vi "slow_control_alpha.vi"() -> ()   [LabVIEW 2018]
uses:
  <instrlib>/Lake Shore 335/Lake Shore 335.lvlib
  <instrlib>/CAEN PSM/CAEN PSM.lvlib
panel:
  in  "stop":bool
  out "Anode resets in":string
  out "CAEN 1 \nVoltages":dbl[](array[numeric])
  out "Started up?":bool
  out "Try 2 Inside loop":dbl[][](array[numeric])
  in  "Read T every N cycles":i32=2
  out "Time until next cycle":dbl
  in  "Time per cycle (s)":i32=2 caption="Time Target (s)"
  in  "input cluster":errorcluster
  in  "Allows tabs on \nfront panel":T1(tab)
  in  "COM-port NI-box":refnum<visa-resource-name>
  in  "COM-port LakeShore":refnum<visa-resource-name>
  in  "ID Query":bool=TRUE
  in  "COM-port CAEN 1":refnum<visa-resource-name>
  in  "COM-port CAEN 2":refnum<visa-resource-name>
  in  "Ignore Initialization Errors":bool caption="Ignore init. errors?"
  out "LakeShore status":bool
  out "NI-box status":bool
  out "CAEN 1 status":bool
  out "CAEN 2 status":bool
  out "Initialization status":bool
  in  "VSet":dbl[](array[numeric])
  in  "IMax (uA)":dbl[](array[numeric])
  in  "VMax (V)":dbl[](array[numeric])
  out "Cathode":dbl(knob) scale=0.0..5000.0
  out "Anode":dbl(knob) scale=0.0..4000.0
  out "PMT 2":dbl(knob) scale=0.0..1000.0
  out "PMT 1":dbl(knob) scale=1.0..1000.0
  in  "Read V every N cycles":i16=120
  out "CAEN 1\nVmon (V)":dbl[](array[numeric])
  out "CAEN 1\nIMon (uA)":dbl[](array[numeric])
  in  "Reset anode":bool=TRUE
  in  "Kill every Y minutes":i32
  in  "Keep off for X seconds":i32
  out "Total cycles in Anode Reset Routine":i32
  out "Current modulated cycle number":i32
  out "VSet killed":bool
  out "VSet applied":bool
  # "<- Proof of concept for New/Old T + New P"
  # "PMT 1"
  # "PMT 2"
  # "Anode"
  # "Cathode"
  # "seconds"
  # "Connection settings"
  # "Lakeshore settings"
  # "Pressure correction settings"
  # "Pressure correction factors go here.\nPrecisely, offsets and multiplication factors\nin the voltages passed from the pressure-\nsensors to the NI-box."
  # "Might need to split up NI-box com port.\nPreferable to task it with measuring T\nand P seperately.\nPerhaps need to set task per single channel."
  # "Alarm indicators"
  # "CAEN 1"
  # "Data"
  # "PMT 1"
  # "PMT 1"
  # "PMT 2"
  # "PMT 2"
  # "Arrays from CAEN 2 go here"
  # "Anode"
  # "Anode"
  # "Cathode"
  # "Cathode"
  # "Settings"
  # "CAEN 1"
  # "CAEN 2"
  # "PMT 1"
  # "PMT 2"
  # "Anode"
  # "CAEN 2"
  # "Cathode"
  # "PMT 1"
  # "PMT 2"
  # "Anode"
  # "Cathode"
  # "Needle gauges or other displays go here"
  # "PMT 1"
  # "PMT 2"
  # "Anode"
  # "Cathode"
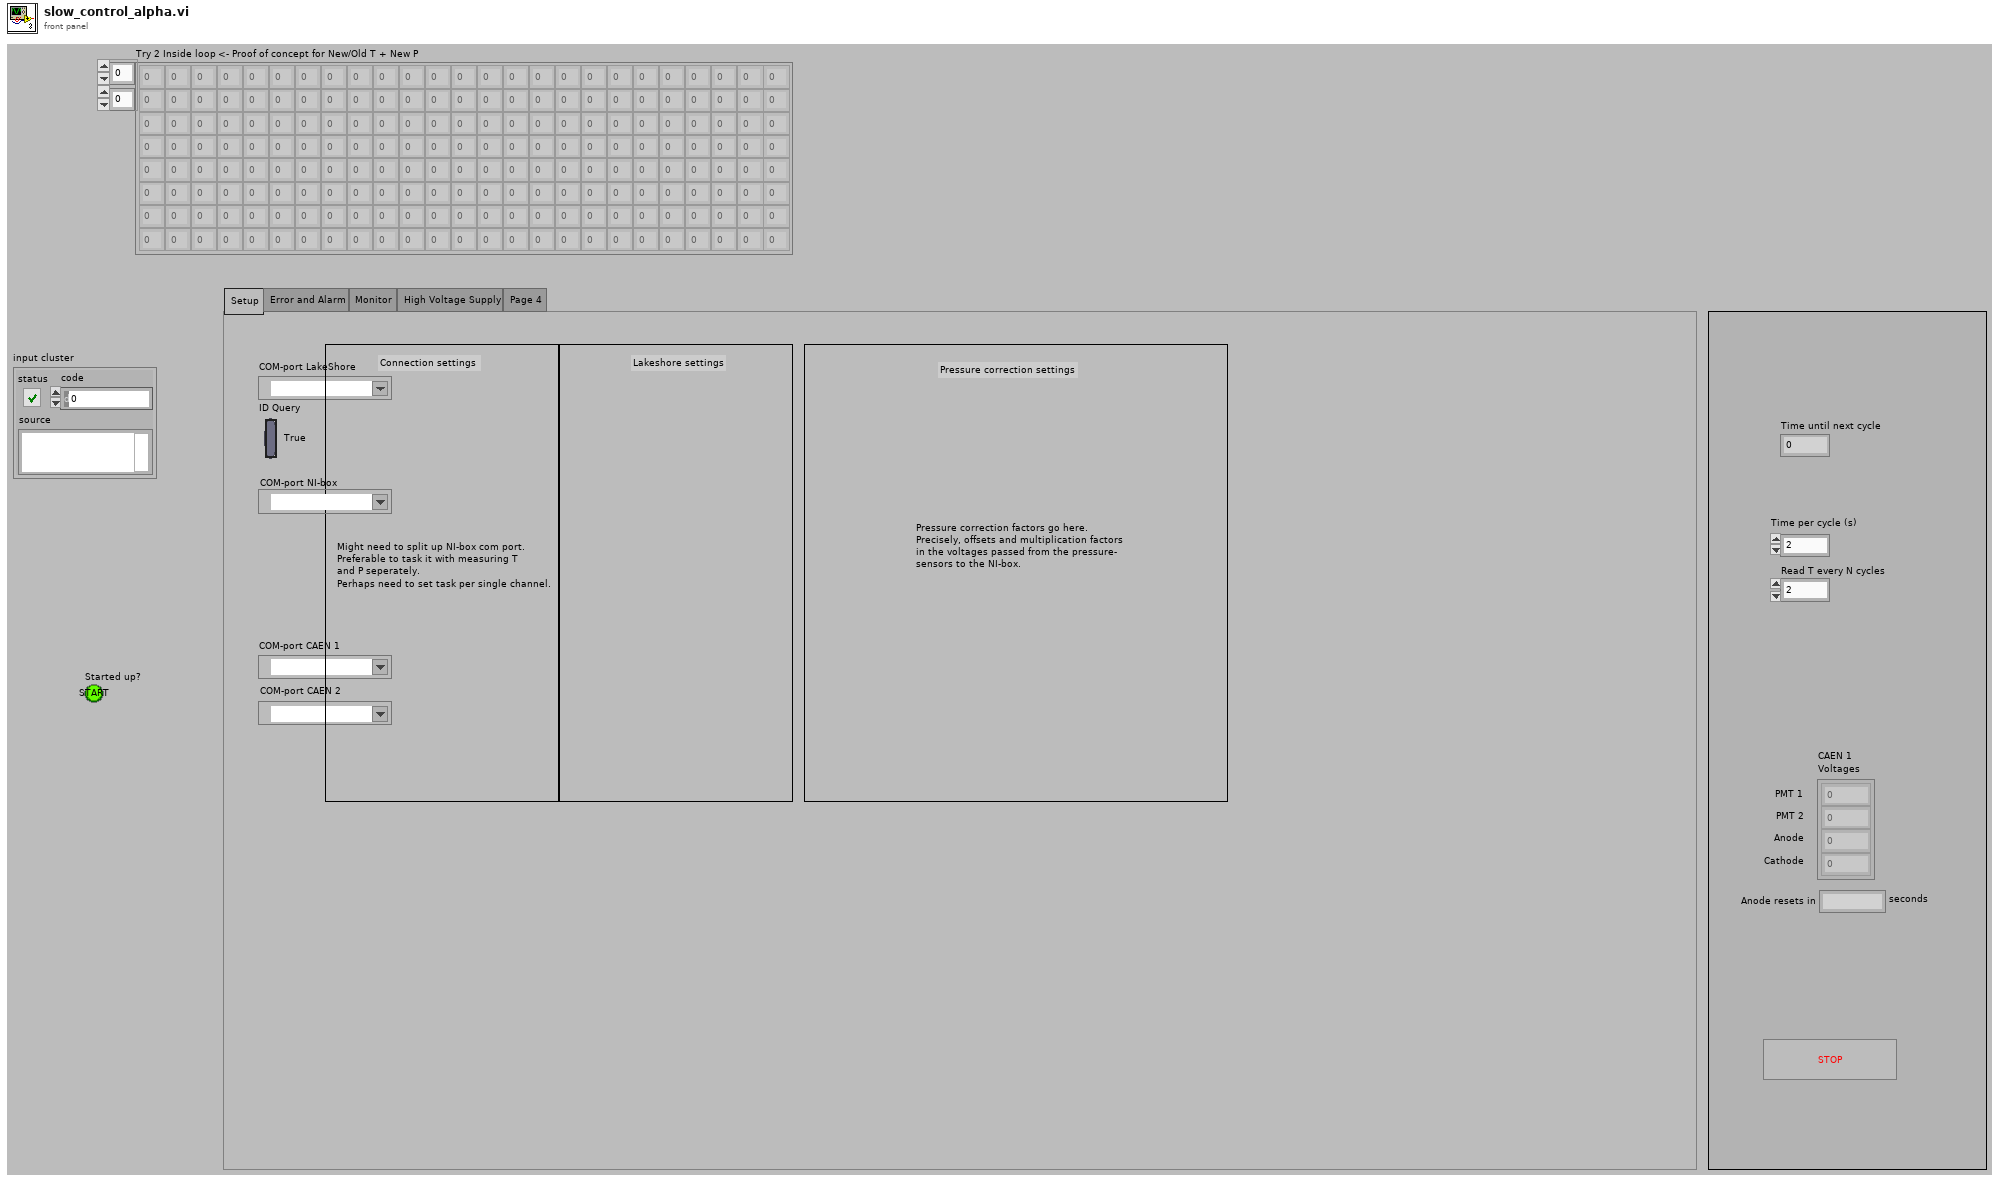
[diagram p1: front panel]
types:
  T1 = enum32{"Setup", "Error and Alarm", "Monitor", "High Voltage Supply", "Page 4"}
  T2 = cluster{"Flow Control":u16, "Stop Bits":u16, "Data Bits":u16, "Parity":u16, "Baud Rate":u32}
  T3 = cluster{"VISA resource name out":refnum<visa-resource-name>, "error out":errorcluster}
  T4 = cluster{"VMax (V)":dbl[], "IMax (uA)":dbl[], "VSet":dbl[]}
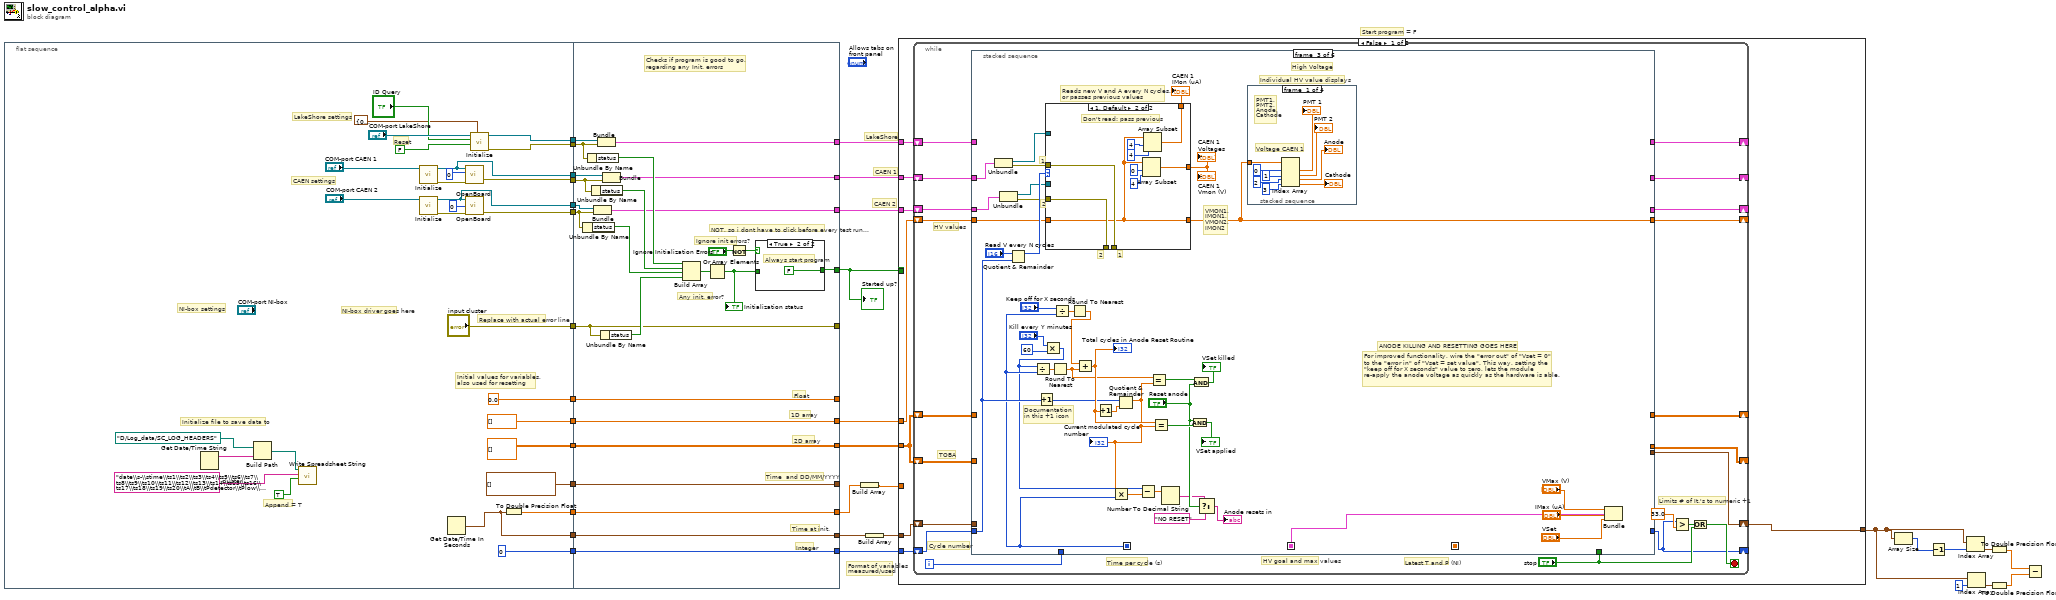
[diagram p0: block diagram]
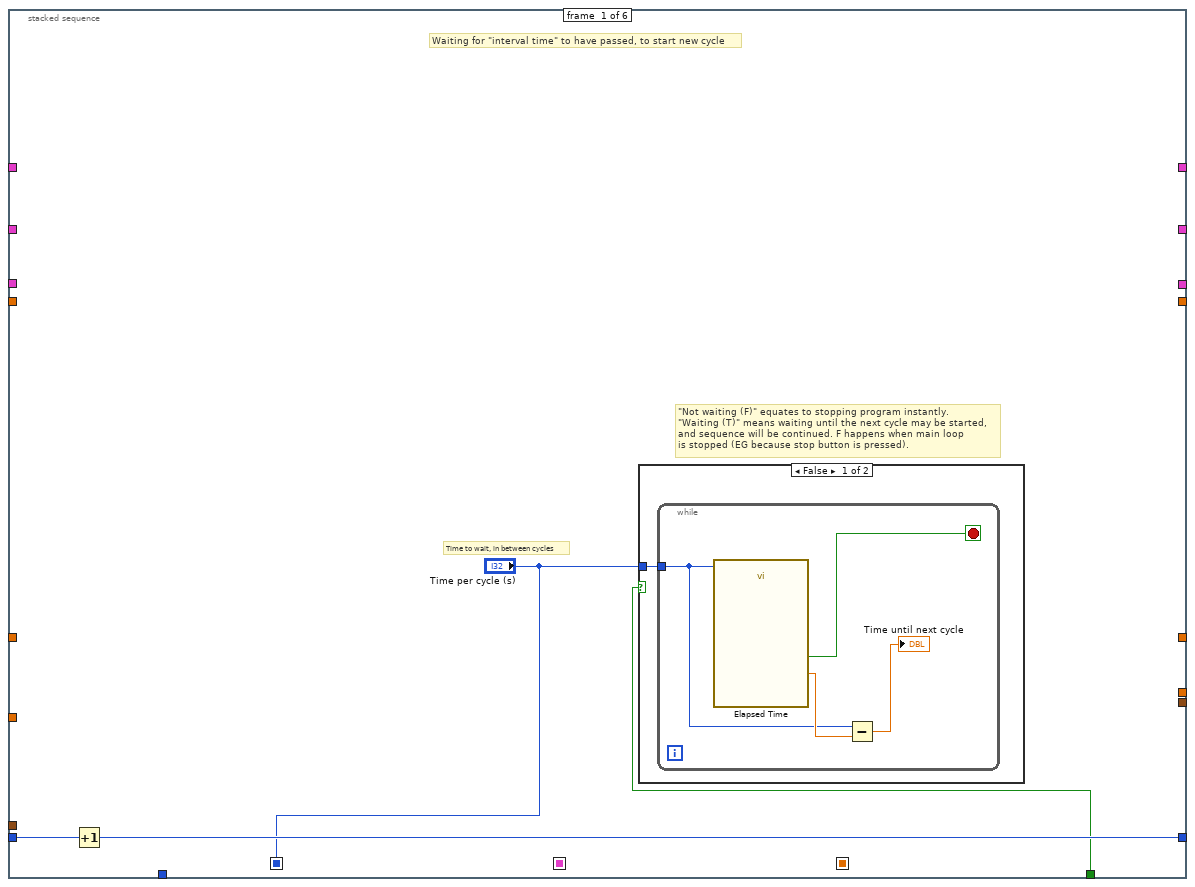
[diagram p2: hidden frame]
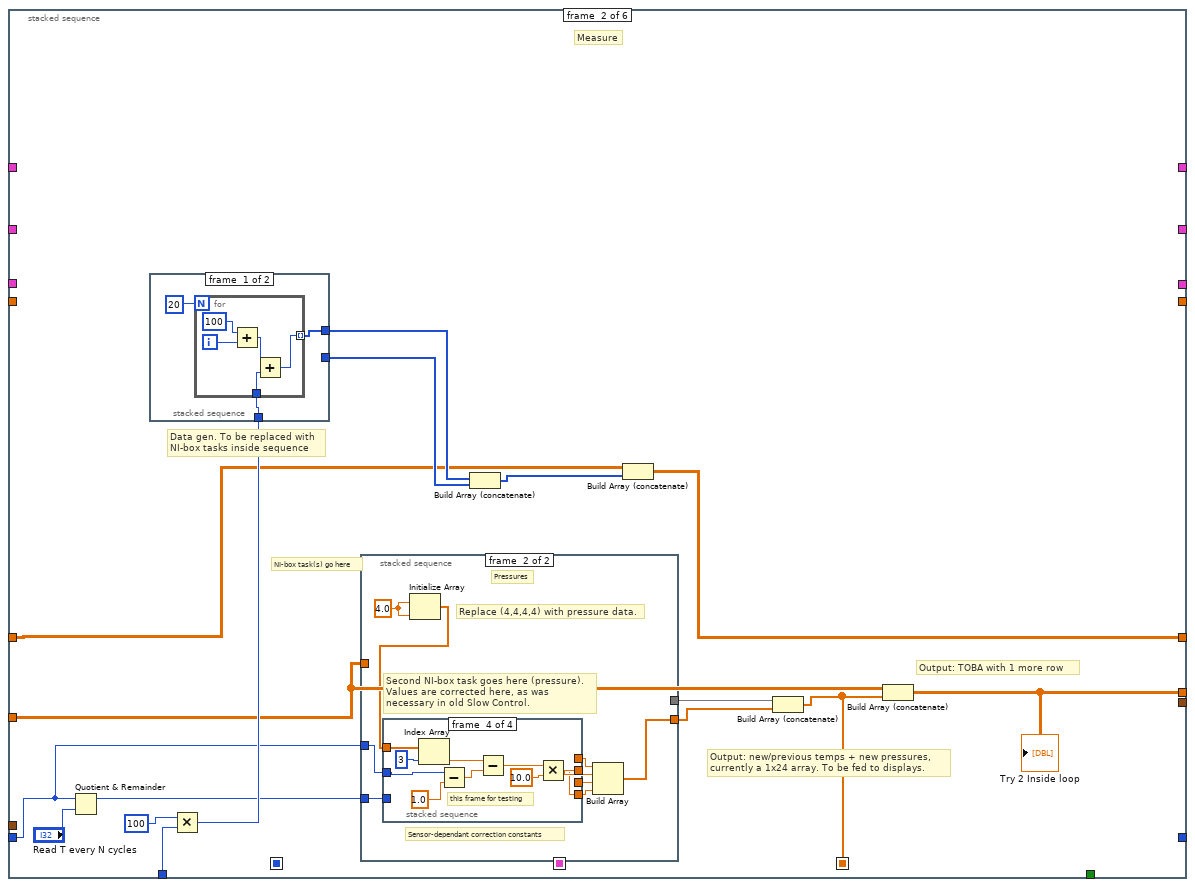
[diagram p4: hidden frame]
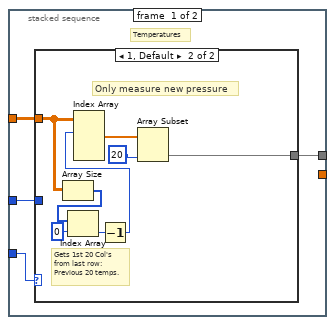
[diagram p5: hidden frame]
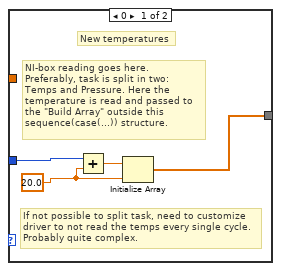
[diagram p6: hidden frame]
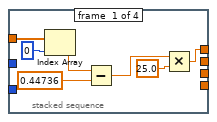
[diagram p7: hidden frame]
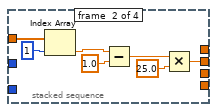
[diagram p8: hidden frame]
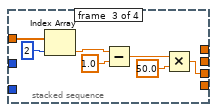
[diagram p9: hidden frame]
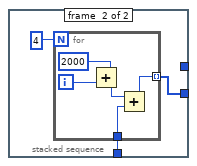
[diagram p10: hidden frame]
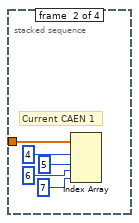
[diagram p11: hidden frame]
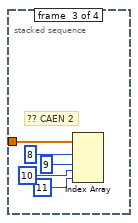
[diagram p12: hidden frame]
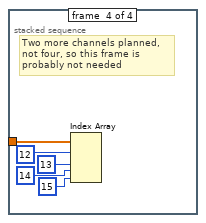
[diagram p13: hidden frame]
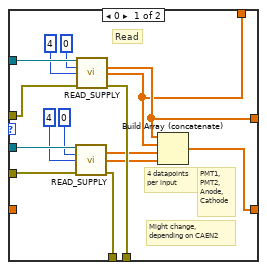
[diagram p14: hidden frame]
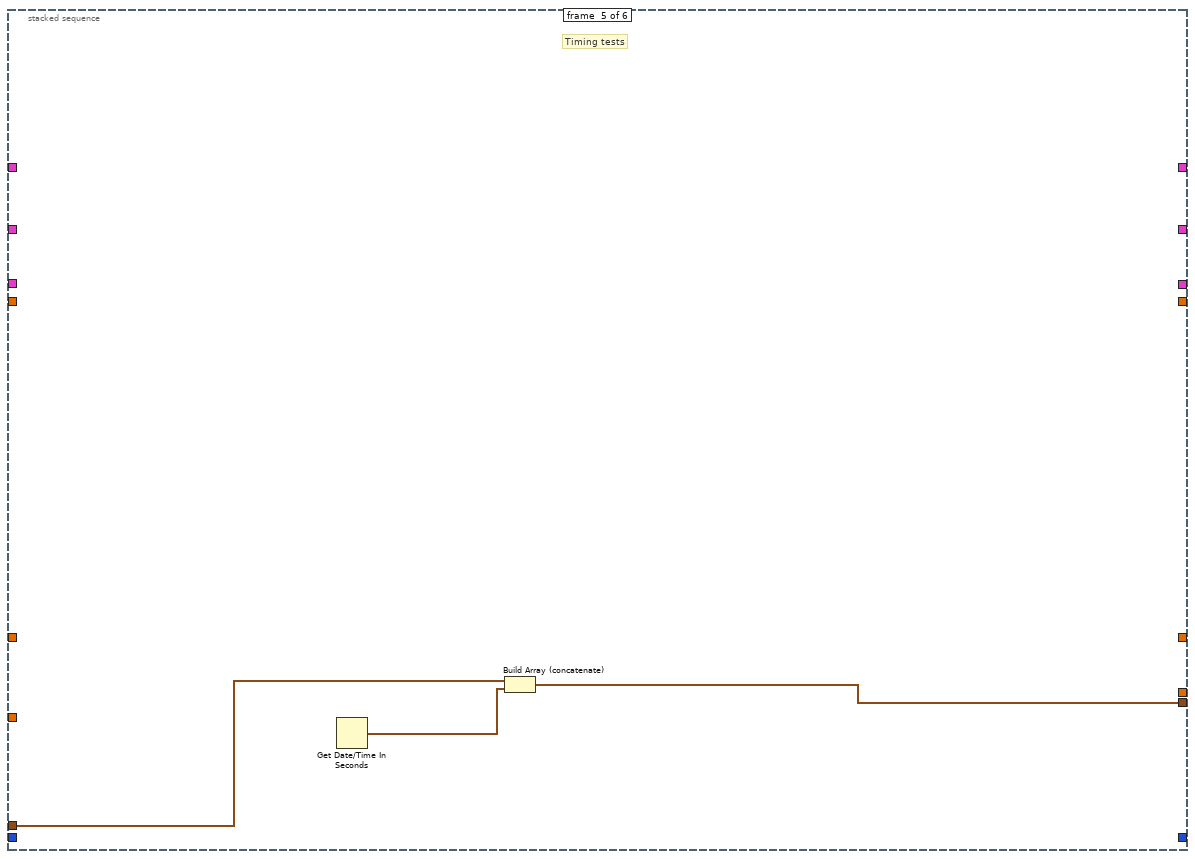
[diagram p16: hidden frame]
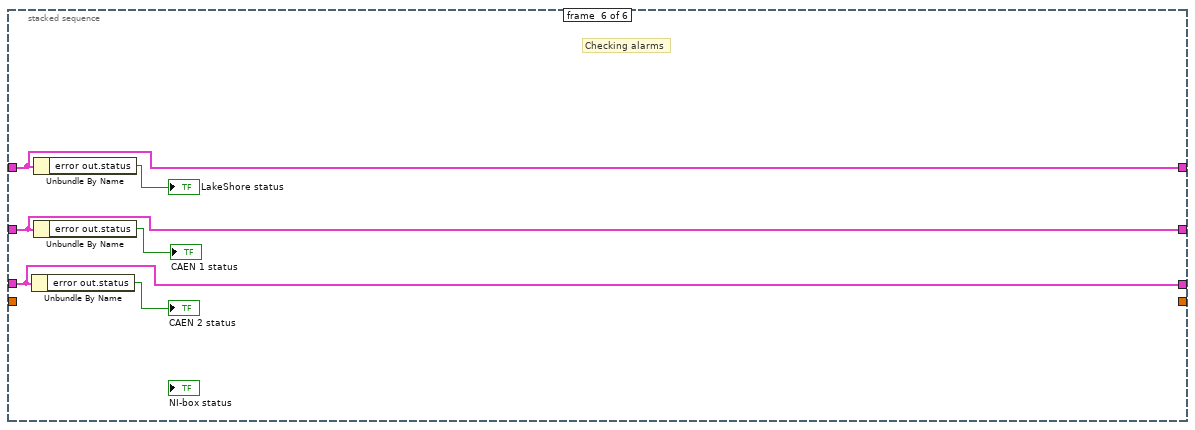
[diagram p17: hidden frame]
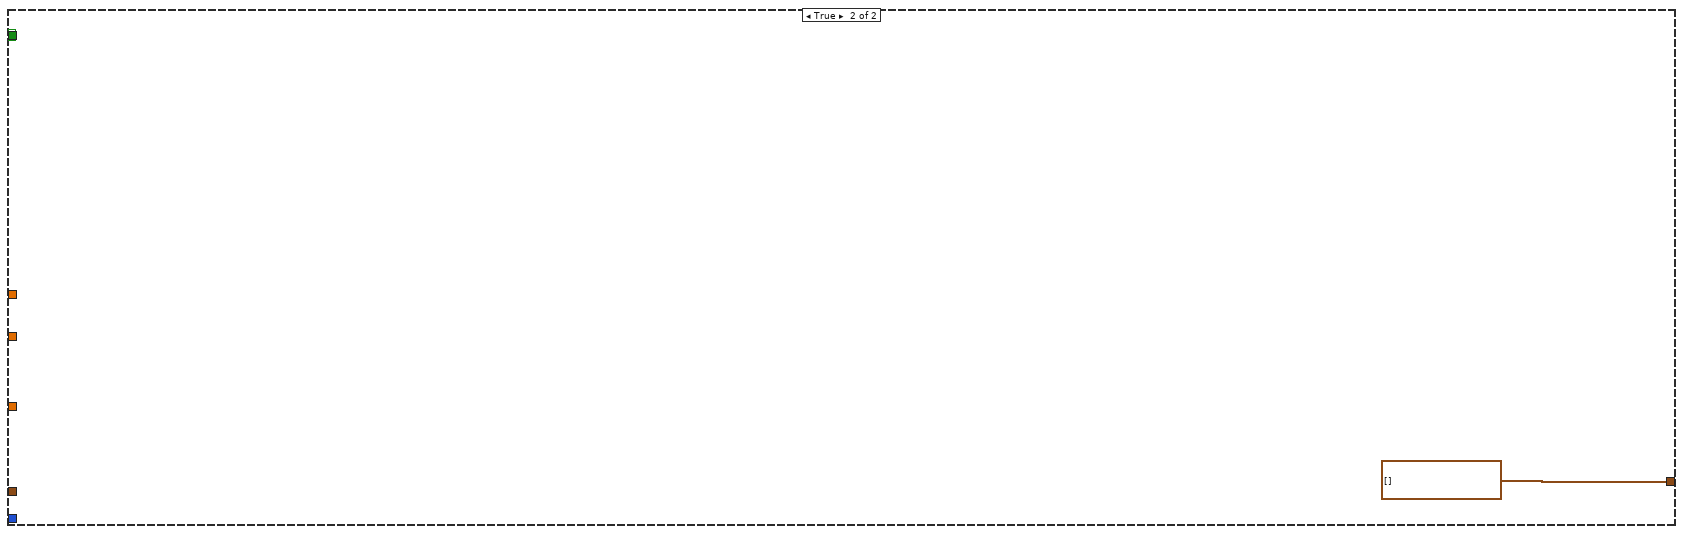
[diagram p18: hidden frame]
diagram:
  # "Start program = F"
  # "CAEN 2"
  # "CAEN 1"
  # "LakeShore"
  # "Format of variables\nmeasured/used"
  n1 = flat-sequence {
    tunnel: [w59] -> w33
    tunnel: [w58] -> w32
    tunnel: [w54] -> w31
    tunnel: [w53] -> w30
    tunnel: ["input cluster"] -> w29
    tunnel: [0.0] -> w28
    tunnel: [dbl[] []] -> w27
    tunnel: [dbl[][] []] -> w26
    tunnel: [timestamp[] []] -> w25
    tunnel: [0] -> w24
    tunnel: [w46] -> w23
    tunnel: [w39] -> w15
    tunnel: [w35] -> w4
    tunnel: [w34] -> w3
    tunnel: w33 -> [w75]
    tunnel: w32 -> [w74]
    tunnel: w31 -> [w72]
    tunnel: w30 -> [w71]
    tunnel: w29 -> [w77]
    tunnel: [w84] -> w1
    tunnel: [w82] -> _
    tunnel: w28 -> [w82]
    tunnel: [w81] -> w22
    tunnel: w27 -> [w81]
    tunnel: [w80] -> w20
    tunnel: w26 -> [w80]
    tunnel: [w79] -> _
    tunnel: w25 -> [w79]
    tunnel: [w78] -> w21
    tunnel: w24 -> [w78]
    tunnel: [w77] -> _
    tunnel: [w76] -> w17
    tunnel: w23 -> [w76]
    tunnel: [w73] -> w19
    tunnel: [w70] -> w18
    tunnel: [w67] -> w14
    tunnel: w15 -> [w67]
    tunnel: w4 -> [w65]
    tunnel: w3 -> [w64]
    tunnel: [w63] -> w2
    frame #0 {
      # "Append = T"
      # "Change to fit order of data in cluster"
      # "Initialize file to save data to"
      # "Initial values for variables,\nalso used for resetting"
      # "Replace with actual error line"
      # "NI-box driver goes here"
      # "NI-box settings"
      # "CAEN settings"
      # "Reset"
      # "LakeShore settings"
      n2 = Get Date/Time String() -> (date string=w42:string)  [unwired: 3 in, 1 out]
      n3 = Build Path(base path=path "D:/Log_data/SC_LOG_HEADERS", name or relative path=w42) -> (appended path=w45:path)
      n4 = call <vilib>:"Write Spreadsheet String.vi"("append to file? (new file:F)"=TRUE, "spreadsheet string"="date\\s-\\stime\\ts1\\ts2\\ts3\\ts4\\ts5\\ts6\\ts7\\ts8\\ts9\\ts10\\ts11\\ts12\\ts13\\ts14\\ts15\\ts16\\ts17\\ts18\\ts19\\ts20\\tA\\tB\\tPdetector\\tPlow\\tPhigh\\tFlow\\tHeater\\tSetpoint\\tCapacitance\\tTimestamp\\tInterval\\tLevel\\tV_PMT1\\tV_PMT2\\tV_Anode\\tV_cathode\\tI_PMT1\\tI_PMT2\\tI_Anode\\tI_cathode\\t\\r\\n", "file path (dialog if empty)"=w45) -> ()  [unwired: 7 in, 2 out]
      n5 = call <instrlib>:"Initialize.vi"("VISA resource name"="COM-port CAEN 1") -> ("error out"=w55:errorcluster, "VISA resource name out"=w54:refnum<visa-resource-name>)  [unwired: 9 in]
      n6 = call <instrlib>:"Initialize.vi"("VISA resource name"="COM-port CAEN 2") -> ("error out"=w36:errorcluster, "VISA resource name out"=w35:refnum<visa-resource-name>)  [unwired: 9 in]
      n7 = Get Date/Time In Seconds() -> (seconds since 1Jan1904=w39:timestamp)
      n8 = call <instrlib>:"OpenBoard.vi"("error in (no error)"=w55, "Board Address"=0, "VISA resource name"=w54) -> ("error out"=w53:errorcluster)  [unwired: 7 in, 1 out]
      n9 = call <instrlib>:"OpenBoard.vi"("error in (no error)"=w36, "Board Address"=u8 0, "VISA resource name"=w35) -> ("error out"=w34:errorcluster)  [unwired: 7 in, 1 out]
      n10 = call <instrlib>:"Initialize.vi"("Serial Configuration"=T2 {"Flow Control"=0, "Stop Bits"=10, "Data Bits"=7, "Parity"=1, "Baud Rate"=57600}, "Reset (True)"=FALSE ("Reset (LakeShore)"), "ID Query (True)"="ID Query", "VISA resource name"="COM-port LakeShore") -> ("error out"=w58:errorcluster, "VISA resource name out"=w59:refnum<visa-resource-name>)  [unwired: 6 in]
      n11 = To Double Precision Float(number=w39) -> (double precision float=w46:dbl)
    }
    frame #1 {
      # "NOT, so i dont have to click before every test run..."
      # "Time at init."
      # "Integer"
      # "Time  and DD/MM/YYYY"
      # "2D array"
      # "1D array"
      # "Float"
      # "Checks if program is good to go,\nregarding any Init. errors"
      # "Ignore init errors?"
      # "Any init. error?"
      n12 = Unbundle By Name(w64) -> ("status"=w66:bool)
      n13 = Unbundle By Name(w74) -> ("status"=w85:bool)
      n14 = Unbundle By Name(w71) -> ("status"=w87:bool)
      n15 = Bundle("VISA resource name out"=w65, "error out"=w64) -> (w63:T3)  [unwired: 1 in]
      n16 = Bundle("VISA resource name out"=w75, "error out"=w74) -> (w73:T3)  [unwired: 1 in]
      n17 = Unbundle By Name(w77) -> ("status"=w86:bool)
      n18 = Bundle("VISA resource name out"=w72, "error out"=w71) -> (w70:T3)  [unwired: 1 in]
      n19 = Build Array(w85, w87, w86, w66) -> (w88:bool[])
      n20 = Or Array Elements(Boolean array=w88) -> (logical OR=w83:bool)
      "Initialization status" <- w83
      n21 = Not(x="Ignore Initialization Errors") -> (.not. x?=w68:bool)
      n22 = case shown="True" w68 {
        tunnel: [w89 FALSE] -> w84
        tunnel: w83 -> [w89 _]
        frame False {
          # "Only start if no errors"
        }
        frame True {
          # "Always start program"
        }
      }
    }
  }
  n23 = Build Array(w17) -> (w16:dbl[])
  n24 = Build Array(w14) -> (w13:timestamp[])
  n25 = case shown="False" w1 {
    selector: w1 -> [_ w314]
    tunnel: [_ w314] -> _
    tunnel: w22 -> [w93 _]
    tunnel: w21 -> [w98 _]
    tunnel: w20 -> [w97 _]
    tunnel: w19 -> [w91 _]
    tunnel: w18 -> [w94 _]
    tunnel: w16 -> [_ _]
    tunnel: w13 -> [w96 _]
    tunnel: [w95 timestamp[] []] -> w9
    tunnel: w2 -> [w92 _]
    frame False {
      n26 = while {
        shift-right: [w107] -> _
        shift-left: w98 -> [w119]
        shift-right: [w113] -> _
        shift-left: w97 -> [w112]
        shift-right: [w110] -> _
        shift-left: w97 -> [w111]
        shift-right: [w108] -> w95
        shift-left: w96 -> [w109]
        shift-right: [w101] -> _
        shift-left: w94 -> [w106]
        shift-right: [w99] -> _
        shift-left: w93 -> [w105]
        shift-right: [w100] -> _
        shift-left: w92 -> [w104]
        shift-right: [w102] -> _
        shift-left: w91 -> [w103]
        i -> [w114]
        stop <- w115 stop-if-true
        # "Time per cycle (s)"
        # "Cycle number"
        # "HV goal and max values"
        # "HV values"
        # "TOBA"
        # "Latest T and P (NI)"
        # "Limits # of It.'s to numeric +1"
        n27 = stacked-sequence {
          seq-local: [_ w131 _ _ _ _] -> [_ _ _ _ _ _]
          seq-local: [_ _ w240 _ _ _] -> [_ _ _ _ _ _]
          seq-local: ["Time per cycle (s)" _ _ _ _ _] -> [_ _ w218 _ _ _]
          tunnel: [w122 _ _ _ _ _] -> w107
          tunnel: "stop" -> [w121 _ _ _ _ _]
          tunnel: w119 -> [w123 w129 w235 _ _ _]
          tunnel: w114 -> [_ w130 _ _ _ _]
          tunnel: w112 -> [_ w136 _ _ _ _]
          tunnel: [_ w140 _ _ _ _] -> w113
          tunnel: w111 -> [_ w132 _ _ _ _]
          tunnel: [_ w133 _ _ _ _] -> w110
          tunnel: w109 -> [_ _ _ _ w305 _]
          tunnel: [_ _ _ _ w304 _] -> w108
          tunnel: w106 -> [_ _ w253 _ _ w309]
          tunnel: w105 -> [_ _ w250 _ _ _]
          tunnel: w104 -> [_ _ w249 _ _ w308]
          tunnel: w103 -> [_ _ _ _ _ w307]
          tunnel: [_ _ _ _ _ w307] -> w102
          tunnel: [_ _ _ _ _ w309] -> w101
          tunnel: [_ _ _ _ _ w308] -> w100
          tunnel: [_ _ w246 _ _ _] -> w99
          frame #0 {
            # "Time to wait, in between cycles"
            # "\"Not waiting (F)\" equates to stopping program instantly.\n\"Waiting (T)\" means waiting until the next cycle may be started,\nand sequence will be continued. F happens when main loop \nis stopped (EG because stop button is pressed)."
            # "Waiting for \"interval time\" to have passed, to start new cycle"
            n28 = Increment(x=w123) -> (x+1=w122:i32)
            n29 = case shown="False" w121 {
              tunnel: "Time per cycle (s)" -> [w124 _]
              frame False {
                n30 = while {
                  tunnel: w124 -> [w126]
                  stop <- w128 stop-if-true
                  n31 = call "Elapsed Time"("Time Target (s)"=w126) -> ("Elapsed Time (s)"=w127:dbl, "Time has Elapsed"=w128:bool)  [unwired: 11 in, 6 out]
                  n32 = Subtract(x=w126, y=w127) -> (x-y=→"Time until next cycle":dbl)
                }
              }
              frame True {
              }
            }
          }
          frame #1 {
            # "Output: TOBA with 1 more row"
            # "Output: new/previous temps + new pressures,\ncurrently a 1x24 array. To be fed to displays."
            # "NI-box task(s) go here"
            # "Data gen. To be replaced with\nNI-box tasks inside sequence"
            # "Measure"
            n33 = Quotient & Remainder(x=w129, y="Read T every N cycles") -> (x-y*floor(x/y)=w137:i32)  [unwired: 1 out]
            n34 = Multiply(x=100, y=w130) -> (x*y=w143:i32)
            n35 = stacked-sequence {
              tunnel: [w201 _] -> w142
              tunnel: [_ w209] -> w141
              tunnel: w143 -> [w200 w208]
              frame #0 {
                n36 = for {
                  N: 20 -> [_]
                  tunnel: [w203] -> w201 mode=indexing
                  tunnel: w200 -> [w205]
                  i -> [w206]
                  n37 = Add(x=100, y=w206) -> (x+y=w204:i32)
                  n38 = Add(x=w204, y=w205) -> (x+y=w203:i32)
                }
              }
              frame #1 {
                n39 = for {
                  N: 4 -> [_]
                  tunnel: [w212] -> w209 mode=indexing
                  tunnel: w208 -> [w211]
                  i -> [w214]
                  n40 = Add(x=2000, y=w214) -> (x+y=w213:i32)
                  n41 = Add(x=w213, y=w211) -> (x+y=w212:i32)
                }
              }
            }
            n42 = stacked-sequence {
              tunnel: w137 -> [w148 w162]
              tunnel: [w147 _] -> w135
              tunnel: [_ w165] -> w134
              tunnel: w132 -> [w146 _]
              tunnel: w129 -> [w145 w161]
              frame #0 {
                # "Temperatures"
                n43 = case shown="1, Default" w148 {
                  tunnel: w146 -> [_ w157]
                  tunnel: [w150 w153] -> w147
                  tunnel: w145 -> [w149 _]
                  frame 0 {
                    w151 = 20.0 ("element")
                    # "If not possible to split task, need to customize\ndriver to not read the temps every single cycle.\nProbably quite complex."
                    # "NI-box reading goes here.\nPreferably, task is split in two: \nTemps and Pressure. Here the \ntemperature is read and passed to \nthe \"Build Array\" outside this \nsequence(case(...)) structure."
                    # "New temperatures"
                    n44 = Add(x=w149, y=w151) -> (x+y=w152:dbl)
                    n45 = Initialize Array(w152, w151) -> (w150:dbl[])
                  }
                  frame 1, Default {
                    # "Gets 1st 20 Col's\nfrom last row:\nPrevious 20 temps."
                    # "Only measure new pressure"
                    n46 = Array Size(array=w157) -> (size(s)=w159:i32[])
                    n47 = Index Array(array=w159, index=0) -> (element=w160:i32)
                    n48 = Decrement(x=w160) -> (x-1=w156:i32)
                    n49 = Index Array(array=w157, index (row) #1=w156) -> (element #1=w155:dbl[])  [unwired: 3 in, 1 out]
                    n50 = Array Subset(array=w155, length=20) -> (w153:dbl[])  [unwired: 1 in]
                  }
                }
              }
              frame #1 {
                w164 = 4.0 ("element")
                # "Replace (4,4,4,4) with pressure data."
                # "Second NI-box task goes here (pressure).\nValues are corrected here, as was \nnecessary in old Slow Control."
                # "Sensor-dependant correction constants"
                # "Pressures"
                n51 = Initialize Array(w164, w164) -> (w163:dbl[])
                n52 = stacked-sequence {
                  tunnel: w163 -> [w171 w183 w190 w199]
                  tunnel: [w172 _ _ _] -> w169
                  tunnel: [_ w178 _ _] -> w168
                  tunnel: [_ _ w185 _] -> w167
                  tunnel: [_ _ _ w195] -> w166
                  tunnel: w162 -> [_ _ _ _]
                  tunnel: w161 -> [_ _ _ w191]
                  frame #0 {
                    n53 = Index Array(array=w171, index=0) -> (element=w170:dbl)
                    n54 = Subtract(x=w170, y=0.44736) -> (x-y=w174:dbl)
                    n55 = Multiply(x=w174, y=25.0) -> (x*y=w172:dbl)
                  }
                  frame #1 {
                    n56 = Index Array(array=w183, index=1) -> (element=w177:dbl)
                    n57 = Subtract(x=w177, y=1.0) -> (x-y=w180:dbl)
                    n58 = Multiply(x=w180, y=25.0) -> (x*y=w178:dbl)
                  }
                  frame #2 {
                    n59 = Index Array(array=w190, index=2) -> (element=w184:dbl)
                    n60 = Subtract(x=w184, y=1.0) -> (x-y=w187:dbl)
                    n61 = Multiply(x=w187, y=50.0) -> (x*y=w185:dbl)
                  }
                  frame #3 {
                    # "this frame for testing"
                    n62 = Index Array(array=w199, index=3) -> (element=w194:dbl)
                    n63 = Subtract(x=w191, y=1.0) -> (x-y=w192:dbl)
                    n64 = Subtract(x=w194, y=w192) -> (x-y=w197:dbl)
                    n65 = Multiply(x=w197, y=10.0) -> (x*y=w195:dbl)
                  }
                }
                n66 = Build Array(w169, w168, w167, w166) -> (w165:dbl[])
              }
            }
            n67 = Build Array (concatenate)(w142, w141) -> (w139:i32[])
            n68 = Build Array (concatenate)(w136, w139) -> (w140:dbl[][])
            n69 = Build Array (concatenate)(w135, w134) -> (w131:dbl[])
            n70 = Build Array (concatenate)(w132, w131) -> (w133:dbl[][])
            "Try 2 Inside loop" <- w133
          }
          frame #2 {
            # "VMON1, \nIMON1,\nVMON2,\nIMON2"
            # "For improved functionality, wire the \"error out\" of \"Vset = 0\"\nto the \"error in\" of \"Vset = set value\". This way, setting the\n\"keep off for X seconds\" value to zero, lets the module \nre-apply the anode voltage as quickly as the hardware is able."
            # "ANODE KILLING AND RESETTING GOES HERE"
            # "Documentation\nin this +1 icon"
            # "Individual HV value displays"
            # "1"
            # "2"
            # "1"
            # "2"
            # "Reads new V and A every N cycles,\nor passes previous values"
            # "High Voltage"
            n71 = Unbundle(w253) -> ("VISA resource name out"=w252:refnum<visa-resource-name>, "error out"=w251:errorcluster)
            n72 = Unbundle(w249) -> ("VISA resource name out"=w248:refnum<visa-resource-name>, "error out"=w247:errorcluster)
            n73 = Quotient & Remainder(x="Read V every N cycles", y=w235) -> (x-y*floor(x/y)=w254:i32)  [unwired: 1 out]
            n74 = Increment(x=w235) -> (x+1=w225:i32)
            n75 = Multiply(x="Kill every Y minutes", y=60) -> (x*y=w216:i32)
            n76 = Divide(x=w216, y=w218) -> (x/y=w228:dbl)
            n77 = case shown="1, Default" w254 {
              tunnel: w252 -> [w294 _]
              tunnel: w251 -> [w293 w302]
              tunnel: w250 -> [_ w298]
              tunnel: w248 -> [w290 _]
              tunnel: w247 -> [w289 w303]
              tunnel: [w286 w303] -> _
              tunnel: [w285 w302] -> _
              tunnel: [w284 w298] -> w246
              tunnel: [w283 w299] -> w245
              tunnel: [w282 w295] -> w244
              frame 0 {
                # "Might change, \ndepending on CAEN2"
                # "PMT1,\nPMT2,\nAnode,\nCathode"
                # "4 datapoints\nper input"
                # "Read"
                n78 = call "READ_SUPPLY.vi"("VISA resource name"=w290, "Board address"=u8 0, "NChannels"=u8 4, "error in (no error)"=w289) -> ("VMon values (V)"=w281:dbl[], "IMon values (uA)"=w280:dbl[], "error out"=w286:errorcluster)  [unwired: 9 in]
                n79 = call "READ_SUPPLY.vi"("VISA resource name"=w294, "Board address"=u8 0, "NChannels"=u8 4, "error in (no error)"=w293) -> ("VMon values (V)"=w283:dbl[], "IMon values (uA)"=w282:dbl[], "error out"=w285:errorcluster)  [unwired: 9 in]
                n80 = Build Array (concatenate)(w283, w282, w281, w280) -> (w284:dbl[])
              }
              frame 1, Default {
                # "Don't read: pass previous"
                n81 = Array Subset(array=w298, index=0, length=4) -> (w299:dbl[])
                n82 = Array Subset(array=w298, index=4, length=4) -> (w295:dbl[])
              }
            }
            "CAEN 1 \nVoltages" <- w245
            "CAEN 1\nVmon (V)" <- w245
            "CAEN 1\nIMon (uA)" <- w244
            n83 = Round To Nearest(number=w228) -> (nearest integer value=w220:dbl)
            n84 = Divide(x="Keep off for X seconds", y=w218) -> (x/y=w230:dbl)
            n85 = Round To Nearest(number=w230) -> (nearest integer value=w229:dbl)
            n86 = Add(x=w229, y=w220) -> (x+y=w226:dbl)
            "Total cycles in Anode Reset Routine" <- w226
            n87 = Increment(x=w226) -> (x+1=w234:dbl)
            n88 = Quotient & Remainder(x=w225, y=w234) -> (x-y*floor(x/y)=w219:dbl)  [unwired: 1 out]
            "Current modulated cycle number" <- w219
            n89 = Multiply(x=w219, y=w218) -> (x*y=w217:dbl)
            n90 = Subtract(x=w216, y=w217) -> (x-y=w224:dbl)
            n91 = Equal?(x=w220, y=w219) -> (x = y?=w236:bool)
            n92 = Equal?(x=w226, y=w219) -> (x = y?=w238:bool)
            n93 = Number To Decimal String(number=w224) -> (decimal integer string=w223:string)  [unwired: 1 in]
            n94 = And(x="Reset anode", y=w238) -> (x .and. y?=→"VSet applied":bool)
            n95 = And(x=w236, y="Reset anode") -> (x .and. y?=→"VSet killed":bool)
            n96 = Select(t=w223, s="Reset anode", f="NO RESET") -> (s? t:f=→"Anode resets in":string)
            n97 = stacked-sequence {
              tunnel: w246 -> [w264 w265 w270 w275]
              frame #0 {
                # "Voltage CAEN 1"
                # "PMT1,\nPMT2,\nAnode,\nCathode"
                n98 = Index Array(array=w264, index #1=0 ("index"), index #2=1 ("index"), index #3=2 ("index"), index #4=3 ("index")) -> (element #1=→"PMT 1":dbl, element #2=→"PMT 2":dbl, element #3=→"Anode":dbl, element #4=→"Cathode":dbl)
              }
              frame #1 {
                # "Current CAEN 1"
                n99 = Index Array(array=w265, index #1=4 ("index"), index #2=5 ("index"), index #3=6 ("index"), index #4=7 ("index")) -> ()  [unwired: 4 out]
              }
              frame #2 {
                # "?? CAEN 2"
                n100 = Index Array(array=w270, index #1=8 ("index"), index #2=9 ("index"), index #3=10 ("index"), index #4=11 ("index")) -> ()  [unwired: 4 out]
              }
              frame #3 {
                # "Two more channels planned, \nnot four, so this frame is\nprobably not needed"
                n101 = Index Array(array=w275, index #1=12 ("index"), index #2=13 ("index"), index #3=14 ("index"), index #4=15 ("index")) -> ()  [unwired: 4 out]
              }
            }
            n102 = Bundle("VMax (V)"="VMax (V)", "IMax (uA)"="IMax (uA)", "VSet"="VSet") -> (w240:T4)  [unwired: 1 in]
          }
          frame #3 {
            # "Reset anode"
          }
          frame #4 {
            # "Timing tests"
            n103 = Get Date/Time In Seconds() -> (seconds since 1Jan1904=w306:timestamp)
            n104 = Build Array (concatenate)(w305, w306) -> (w304:timestamp[])
          }
          frame #5 {
            # "Checking alarms"
            n105 = Unbundle By Name(w308) -> ("error out.status"=→"CAEN 2 status":bool)
            n106 = Unbundle By Name(w307) -> ("error out.status"=→"LakeShore status":bool)
            n107 = Unbundle By Name(w309) -> ("error out.status"=→"CAEN 1 status":bool)
          }
        }
        n108 = Greater?(x=w107, y=33.0 ("x")) -> (0:w117:bool)
        n109 = Or(x=w117, y="stop") -> (x .or. y?=w115:bool)
      }
    }
    frame True {
    }
  }
  n110 = Array Size(array=w9) -> (size(s)=w12:i32)
  n111 = Decrement(x=w12) -> (x-1=w11:i32)
  n112 = Index Array(array=w9, index=w11) -> (element=w10:timestamp)
  n113 = Index Array(array=w9, index=1) -> (element=w7:timestamp)
  n114 = To Double Precision Float(number=w10) -> (double precision float=w6:dbl)
  n115 = To Double Precision Float(number=w7) -> (double precision float=w5:dbl)
  n116 = Subtract(x=w6, y=w5) -> ()  [unwired: 1 out]
  "Started up?" <- w1
